vi "NAND_XOR_SUB.vi"(1 "Boolean 2":bool, 2 "Boolean":bool) -> (0 "Boolean 3":bool)   [LabVIEW 2026]
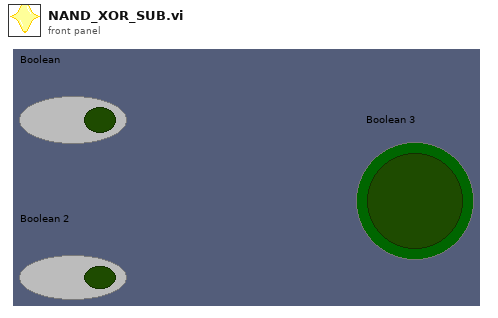
[diagram p1: front panel]
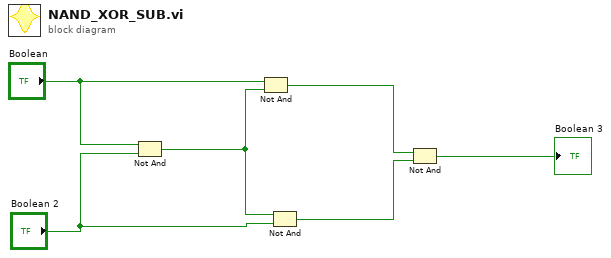
[diagram p0: block diagram]
diagram:
  n1 = Not And(1:"Boolean 2", 2:"Boolean") -> (0:w6:bool)
  n2 = Not And(1:w6, 2:"Boolean") -> (0:w5:bool)
  n3 = Not And(1:"Boolean 2", 2:w6) -> (0:w4:bool)
  n4 = Not And(1:w4, 2:w5) -> (0:→"Boolean 3":bool)
